vi "Write channel array.vi"(8 "error in (no error)":errorcluster, 10 "channel array":T1(array[cluster]), 11 "Y (Complex) (N Ch) in":refnum<class "Y (Complex) (N Ch).lvclass">) -> (0 "error out":errorcluster, 3 "Y (Complex) (N Ch) out":refnum<class "Y (Complex) (N Ch).lvclass">)   [LabVIEW 2017, in "Y (Complex) (N Ch).lvclass"]
uses:
  <vilib>/addons/_NISVFA/_Shared subVIs/Data Objects/Y (Complex) (DBL)/Y (Complex) (N Ch).lvclass
  <vilib>/addons/_NISVFA/_Shared subVIs/Data Objects/Y (Complex) (DBL)/Y (Complex) (N Ch).lvclass/Y (Complex) (N Ch).ctl
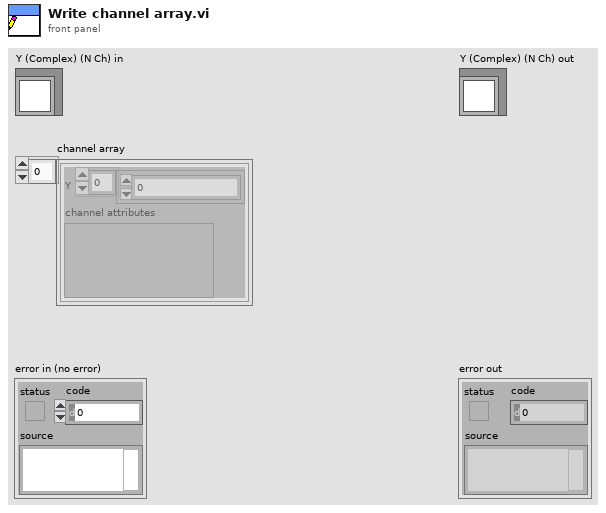
[diagram p1: front panel]
types:
  T1 = cluster{"Y":cdb[], "channel attributes":variant}[]
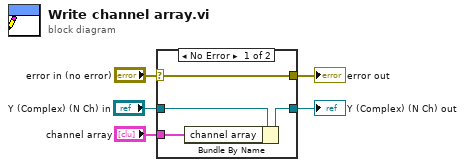
[diagram p0: block diagram]
diagram:
  n1 = case shown="No Error" "error in (no error)" {
    selector: "error in (no error)" -> [w9 w10]
    tunnel: [w9 w10] -> w4
    tunnel: [w6 w11] -> w2
    tunnel: "Y (Complex) (N Ch) in" -> [w8 w11]
    tunnel: "channel array" -> [w7 _]
    frame No Error {
      n2 = Bundle By Name(cluster=w8, "channel array"=w7) -> (w6:refnum<class "Y (Complex) (N Ch).lvclass">)
    }
    frame Error {
    }
  }
  "error out" <- w4
  "Y (Complex) (N Ch) out" <- w2
